vi "FA_StringToSpecialType.vi"(5 "Special Type String":string) -> (2 "Special Type Enum":T1)   [LabVIEW 2013, in "FA_NativeTypes.lvlib"]
doc: "Converts from a Special type string to the enum"
uses:
  FA_NativeTypes.lvlib
  FA_LocalStore API/source/VI Source/FA_LSSpecialTypes.ctl
  FA_LocalStore API/source/VI Source/FA_LocalStore.lvlib
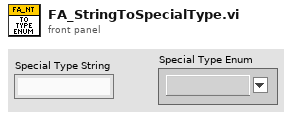
[diagram p1: front panel]
types:
  T1 = typedef "FA_LocalStore.lvlib/FA_LSSpecialTypes.ctl" = string
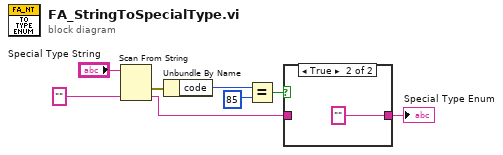
[diagram p0: block diagram]
diagram:
  n1 = Scan From String(input string="Special Type String", default 1=T1 "" ("Special Type")) -> (error out=w6:errorcluster, output 1=w2:T1)  [unwired: 3 in, 2 out]
  n2 = Unbundle By Name(w6) -> ("code"=w5:i32)
  n3 = Equal?(x=w5, y=85) -> (x = y?=w3:bool)
  n4 = case shown="True" w3 {
    tunnel: w2 -> [w9 _]
    tunnel: [w9 T1 "" ("Special Type")] -> w1
    frame False {
    }
    frame True {
    }
  }
  "Special Type Enum" <- w1
